vi "WSVCAP SHL Host LL Interface Instantiated Wrapper.vi"(0 "Message In":string, 11 "error in":errorcluster, 12 "Log (T)":bool=TRUE, 13 "Function":T5, 14 "FPGA":T1) -> (3 "System":T2={"Settings"={"I2C Slave Address"=144, "I2C Clock Rate (Hz)"=20.0, "SPI Clock Rate (Hz)"=50000.0, "RFFE Slave Address"=255, "RFFE Clock Rate (Hz)"=20.0, "Simulate FPGA"=TRUE, "C1 Cap DAC Default"=165, "C2 Cap DAC Default"=165, "C3 Cap DAC Default"=134}, "FPGA Resource"="", "Online"=FALSE, "I2C Wait Ticks"=0, "SPI Wait Ticks"=0, "RFFE Wait Ticks"=0, "FPGA VI Reference (FPGA Mode)"=refnum, "FPGA VI Reference (Sim Mode)"=refnum} {"Settings"."C3 Cap DAC Default" format="0x%02x"; "Settings"."C2 Cap DAC Default" format="0x%02x"; "Settings"."C1 Cap DAC Default" format="0x%02x"; "Settings"."RFFE Clock Rate (Hz)" format="%.0f Hz"; "Settings"."RFFE Slave Address" format="0x%02x"; "Settings"."I2C Clock Rate (Hz)" format="%.0f Hz"; "Settings"."SPI Clock Rate (Hz)" format="%.0f Hz"; "Settings"."I2C Slave Address" format="0x%02x"}, 4 "Message Out":string, 15 "error out":errorcluster)   [LabVIEW 2012]
uses:
  Type Defs/WSVCAP SHL Function Enum.ctl
  Type Defs/WSVCAP SHL Core System Cluster.ctl
  Type Defs/WSVCAP SHL I2C Settings Cluster.ctl
  Type Defs/WSVCAP SHL FPGA VI Reference.ctl
  Type Defs/WSVCAP SHL I2C FPGA Enum.ctl
  user.lib/Utilities/Type Defs/MISC Instance Manager Operation.ctl
  user.lib/Utilities/Type Defs/MISC IO Choice Enum.ctl
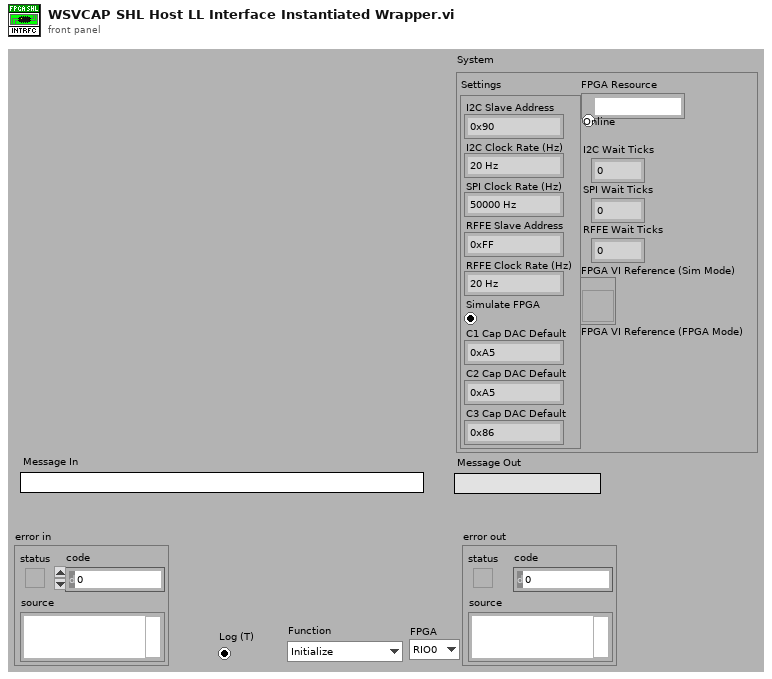
[diagram p1: front panel]
types:
  T1 = typedef "WSVCAP SHL I2C FPGA Enum.ctl" = enum16{"RIO0", "RIO1"}
  T2 = typedef "WSVCAP SHL Core System Cluster.ctl" = cluster{"Settings":T3, "FPGA Resource":tag, "Online":bool, "I2C Wait Ticks":u32, "SPI Wait Ticks":u32, "RFFE Wait Ticks":u32, "FPGA VI Reference (FPGA Mode)":T4, "FPGA VI Reference (Sim Mode)":refnum<vi>}
  T3 = typedef "WSVCAP SHL I2C Settings Cluster.ctl" = cluster{"I2C Slave Address":u8, "I2C Clock Rate (Hz)":dbl, "SPI Clock Rate (Hz)":dbl, "RFFE Slave Address":u8, "RFFE Clock Rate (Hz)":dbl, "Simulate FPGA":bool, "C1 Cap DAC Default":u8, "C2 Cap DAC Default":u8, "C3 Cap DAC Default":u8}
  T4 = typedef "WSVCAP SHL FPGA VI Reference.ctl" = refnum<k20>
  T5 = typedef "WSVCAP SHL Function Enum.ctl" = enum16{"Initialize", "Configure I2C", "Configure RFFE", "Write I2C", "Read I2C", "Write RFFE", "Read RFFE", "Start RFFE Cycle", "Stop RFFE Cycle", "Get Status", "Close"}
  T6 = typedef "MISC IO Choice Enum.ctl" = enum16{"Read", "Write"}
  T7 = typedef "MISC Instance Manager Operation.ctl" = enum16{"Create Instance", "Get Instance ID"}
  T8 = typedef "WSVCAP SHL FPGA Interface Instance Ref Cluster.ctl" = cluster{"Core Instance ID":refnum<vi>, "ST MGR Instance ID":refnum<vi>}
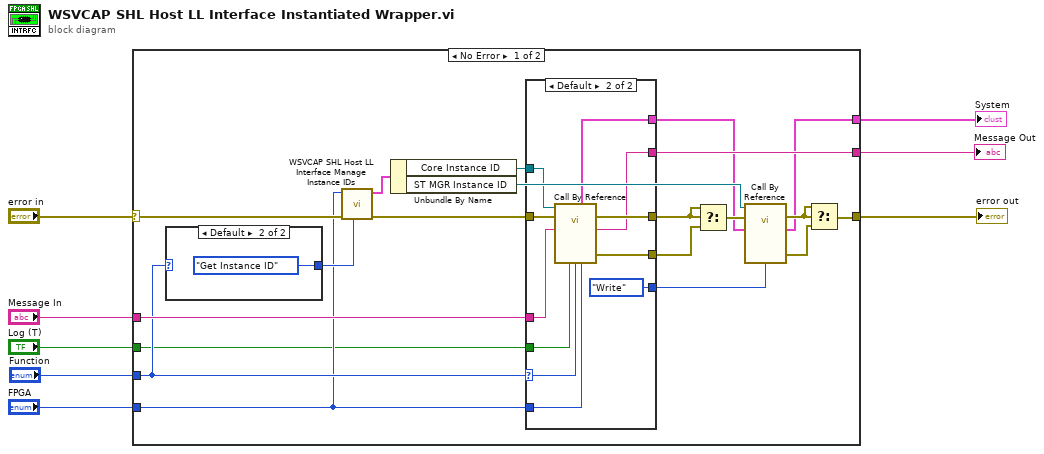
[diagram p0: block diagram]
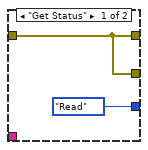
[diagram p2: hidden frame]
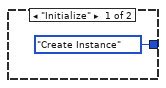
[diagram p3: hidden frame]
diagram:
  n1 = case shown="No Error" "error in" {
    selector: "error in" -> [w28 w44]
    tunnel: [w19 w44] -> w1
    tunnel: "Function" -> [w15 _]
    tunnel: [w13 _] -> w2
    tunnel: "FPGA" -> [w10 _]
    tunnel: [w24 _] -> w3
    tunnel: "Message In" -> [w23 _]
    tunnel: "Log (T)" -> [w9 _]
    frame No Error {
      n2 = case shown="Default" w15 {
        tunnel: [MISC_Instance_Manager_Operation."Create Instance" ("Operation") MISC_Instance_Manager_Operation."Get Instance ID" ("Operation")] -> w16
        frame "Initialize" {
        }
        frame Default {
        }
      }
      n3 = call "WSVCAP SHL Host LL Interface Manage Instance IDs.vi"("Operation"=w16, "error in (no error)"=w28, "FPGA"=w10) -> ("error out"=w27:errorcluster, "Instance IDs"=w22:T8)  [unwired: 7 in]
      n4 = Unbundle By Name(w22) -> ("Core Instance ID"=w21:refnum<vi>, "ST MGR Instance ID"=w12:refnum<vi>)
      n5 = case shown="Default" w15 {
        selector: w15 -> [_ w34]
        tunnel: w27 -> [w29 w41]
        tunnel: [w29 w40] -> w26
        tunnel: [w29 w39] -> w25
        tunnel: [_ w38] -> w24
        tunnel: w23 -> [_ w37]
        tunnel: w21 -> [_ w36]
        tunnel: [_ w35] -> w11
        tunnel: [MISC_IO_Choice_Enum."Read" ("Enum") MISC_IO_Choice_Enum."Write" ("Enum")] -> w14
        tunnel: w10 -> [_ w32]
        tunnel: w9 -> [_ w31]
        frame "Get Status" {
        }
        frame Default {
          n6 = call-by-ref "?"(reference=w36, error in=w41, "Message In"=w37, "Log (T)"=w31, "Function"=w34, "FPGA"=w32) -> (error out=w39:errorcluster, "System"=w35:T2, "Message Out"=w38:string, 15:"error out"=w40:errorcluster)  [unwired: 9 in, 1 out]
        }
      }
      n7 = Select(t=w25, s=w25, f=w26) -> (s? t:f=w20:errorcluster)
      n8 = call-by-ref "?"(reference=w12, error in=w20, "System In"=w11, "Operation (Read)"=w14) -> (error out=w17:errorcluster, "System Out"=w13:T2, 15:"error out"=w18:errorcluster)  [unwired: 12 in, 1 out]
      n9 = Select(t=w17, s=w17, f=w18) -> (s? t:f=w19:errorcluster)
    }
    frame Error {
    }
  }
  "error out" <- w1
  "Message Out" <- w3
  "System" <- w2
